vi "Decay_array.vi"(10 "Power in":dbl, 11 "Array in":dbl[](array[numeric])) -> (2 "Change out":dbl[](array[numeric]), 3 "Array out":dbl[](array[numeric]))   [LabVIEW 2018]
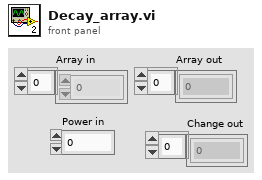
[diagram p1: front panel]
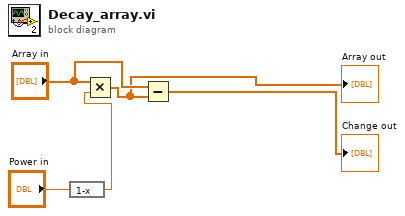
[diagram p0: block diagram]
diagram:
  n1 = expression code="1-x"("Power in") -> (w4:dbl)
  n2 = Multiply(x="Array in", y=w4) -> (x*y=w1:dbl[])
  "Array out" <- w1
  n3 = Subtract(x="Array in", y=w1) -> (x-y=→"Change out":dbl[])
